vi "SUB_COM_NoErrRead_TimeOut.vi"(0 "Timeout Seccond":dbl, 4 "Begin time":dbl, 8 "Find this String":string, 9 "VISA resource name":refnum<visa-resource-name>) -> (1 "concatenated string":string, 3 "Found":bool)   [LabVIEW 2011]
panel:
  out "concatenated string 2":string
  out "Numeric":i32
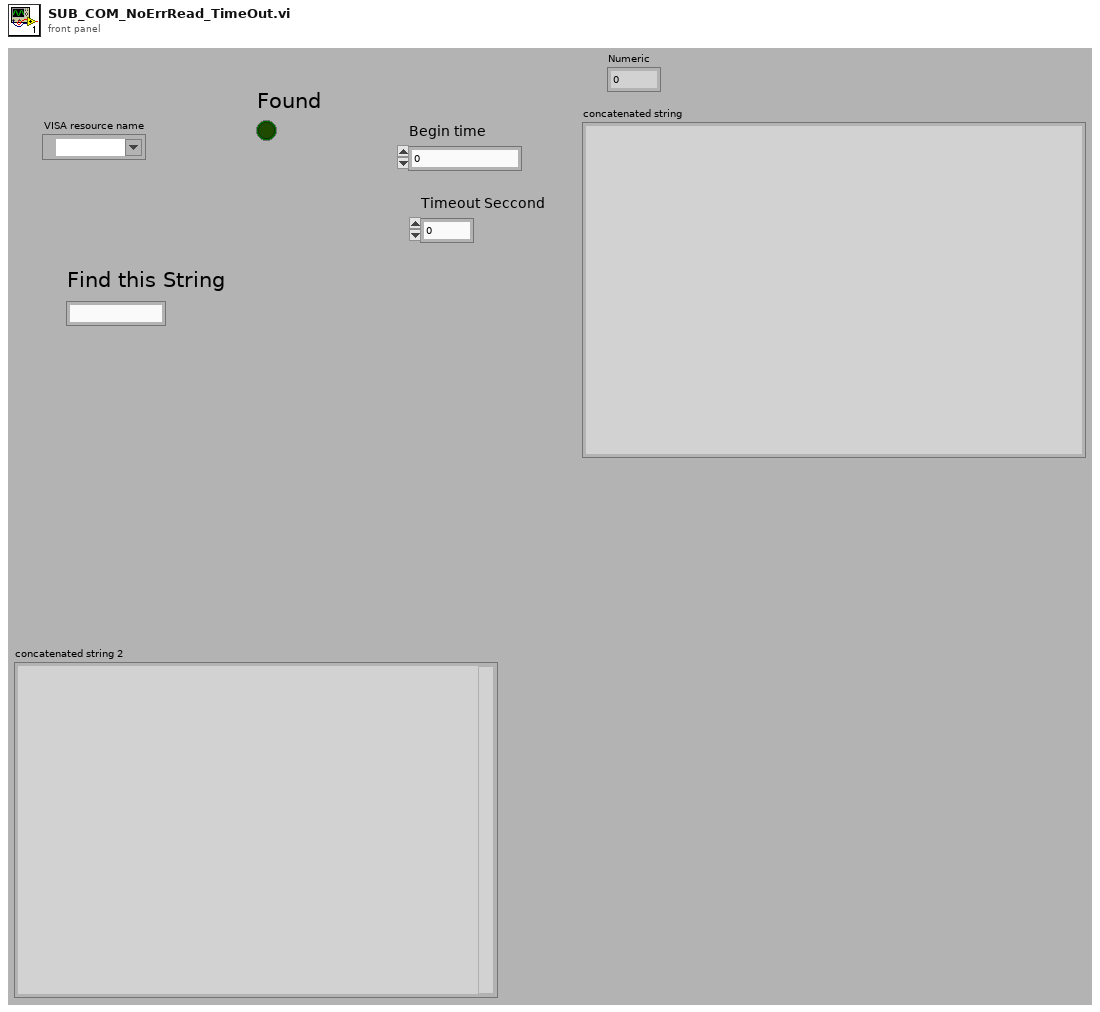
[diagram p1: front panel]
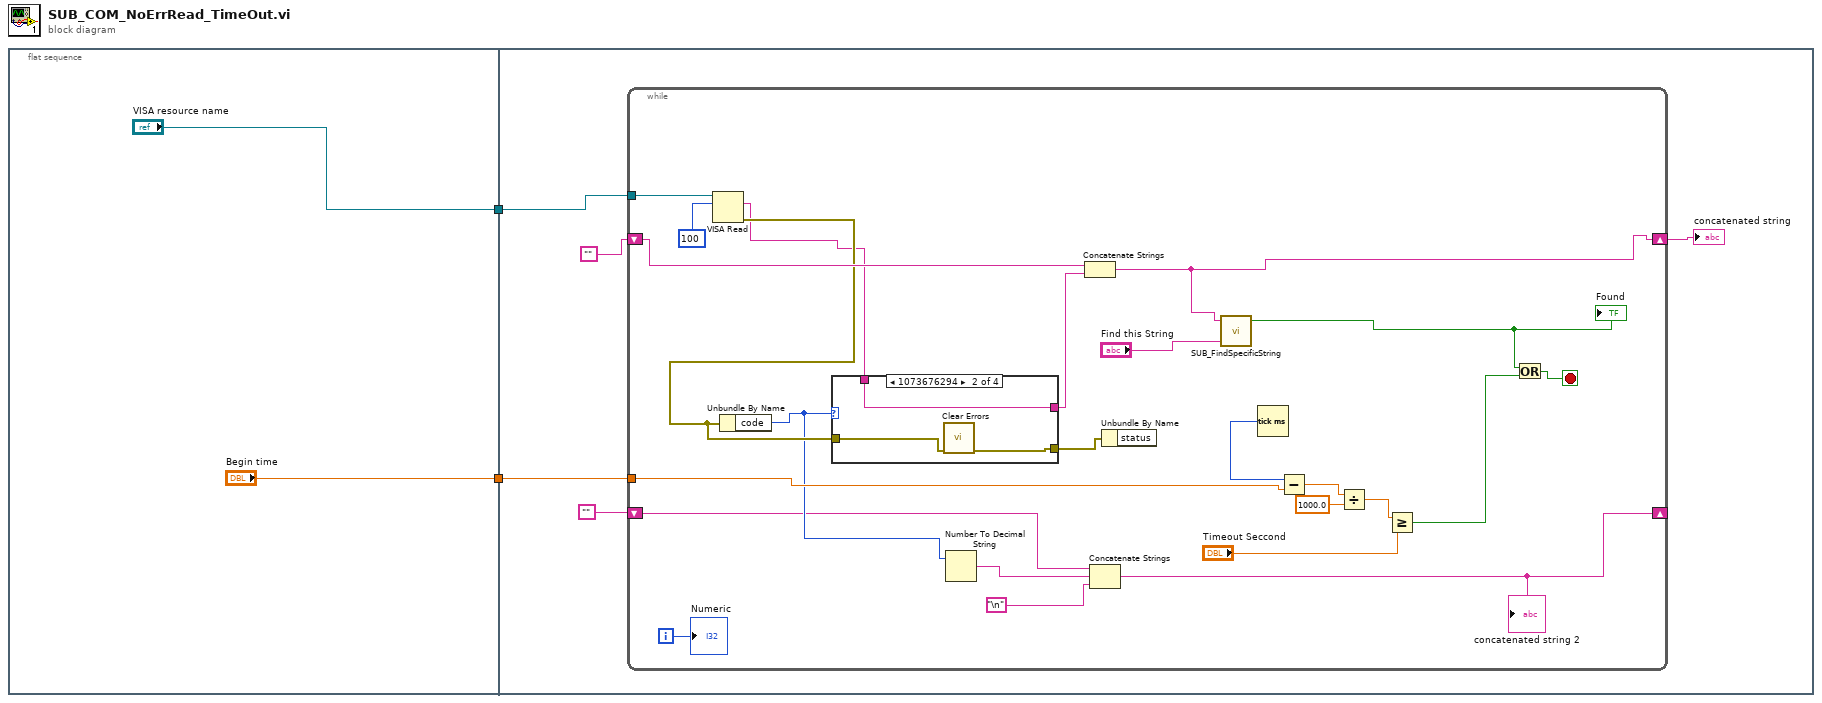
[diagram p0: block diagram]
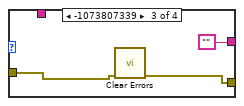
[diagram p3: hidden frame]
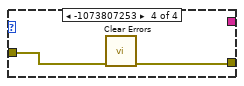
[diagram p4: hidden frame]
diagram:
  n1 = flat-sequence {
    tunnel: ["Begin time"] -> w2
    tunnel: ["VISA resource name"] -> w1
    tunnel: w2 -> [w8]
    tunnel: w1 -> [w6]
    frame #0 {
    }
    frame #1 {
      n2 = while {
        shift-right: [w32] -> w5
        shift-left: "" -> [w33]
        tunnel: w8 -> [w22]
        shift-right: [w17] -> _
        shift-left: "" -> [w16]
        tunnel: w6 -> [w10]
        i -> [w23]
        stop <- w30 stop-if-true
        n3 = VISA Read(VISA resource name=w10, byte count=u32 100 ("bytes to read")) -> (read buffer=w12:string, error out=w20:errorcluster)  [unwired: 1 in, 2 out]
        n4 = Unbundle By Name(w20) -> ("code"=w19:i32)
        n5 = case shown="1073676294" w19 {
          tunnel: w20 -> [w35 w37 w41 w43]
          tunnel: [w35 w36 w40 w42] -> w14
          tunnel: [w34 w38 "" _] -> w13
          tunnel: w12 -> [w34 w38 _ _]
          frame 0, Default {
          }
          frame 1073676294 {
            n6 = call <vilib>:"Clear Errors.vi"("error in (no error)"=w37) -> ("error out"=w36:errorcluster)  [unwired: 6 in]
          }
          frame -1073807339 {
            n7 = call <vilib>:"Clear Errors.vi"("error in (no error)"=w41) -> ("error out"=w40:errorcluster)  [unwired: 6 in]
          }
          frame -1073807253 {
            n8 = call <vilib>:"Clear Errors.vi"("error in (no error)"=w43) -> ("error out"=w42:errorcluster)  [unwired: 6 in]
          }
        }
        n9 = Number To Decimal String(number=w19) -> (decimal integer string=w18:string)  [unwired: 1 in]
        n10 = Concatenate Strings(w33, w13) -> (w32:string)
        n11 = Concatenate Strings(w16, w18, "\n") -> (w17:string)
        "concatenated string 2" <- w17
        n12 = Unbundle By Name(w14) -> ()  [unwired: 1 out]
        n13 = call "SUB_FindSpecificString.vi"("Find this String"="Find this String", "String data"=w32) -> ("Found"=w29:bool)  [unwired: 2 in, 1 out]
        "Found" <- w29
        n14 = Tick Count (ms)() -> (millisecond timer value=w24:u32)
        n15 = Subtract(x=w24, y=w22) -> (x-y=w28:dbl)
        n16 = Divide(x=w28, y=1000.0) -> (x/y=w26:dbl)
        n17 = Greater Or Equal?(x=w26, y="Timeout Seccond") -> (x >= y?=w21:bool)
        n18 = Or(x=w29, y=w21) -> (x .or. y?=w30:bool)
        "Numeric" <- w23
      }
      "concatenated string" <- w5
    }
  }
